vi "Interpret Driver Controls.vi"() -> ()   [LabVIEW 2018]
uses:
  Robot Global Data.vi
  SubSystems/Controllers/Driver Controller/Driver Controller Global.vi
  SubSystems/Drive Train/Drive Train Global.vi
  SubSystems/Lift/Lift Global.vi
  <vilib>/addons/control/pid/pid.llb/PID (DBL).vi
  SubSystems/Controllers/Manipulator Controlller/Manipulator Controller Global.vi
  SubSystems/HAB Climber/HAB Climber Global.vi
  SubSystems/Hatch Panel Intake/Hatch Panel Intake Global.vi
  SubSystems/Cargo Intake/Cargo Intake Global.vi
  <vilib>/addons/control/pid/NI_PID_pid.lvlib
panel:
  in  "Last Move Deadband":u32=500
  in  "Last Time Auto":u32=1171826
  in  "Camera Tracking":T1={"proportional gain (Kc)"=0.06, "integral time (Ti, min)"=0.0, "derivative time (Td, min)"=0.0}
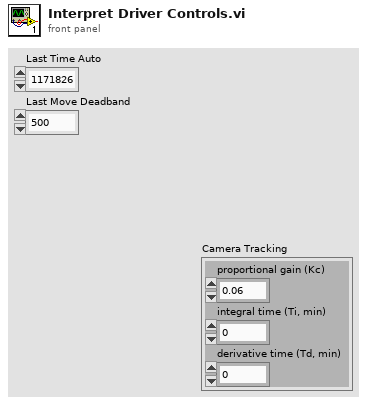
[diagram p1: front panel]
types:
  T1 = cluster{"proportional gain (Kc)":dbl, "integral time (Ti, min)":dbl, "derivative time (Td, min)":dbl}
  T2 = enum16{"Manual", "Hatch Panel Zone 1", "Hatch Panel Zone 2", "Hatch Panel Zone 3", "Cargo Zone 1", "Cargo Zone 2", "Cargo Zone 3", "Cargo Ship Zone"}
  T3 = cluster{"Rollover":dbl, "Yaw":dbl, "Cont Yaw":dbl}
  T4 = enum16{"Hatch Panel Zone 1", "Hatch Panel Zone 2", "Hatch Panel Zone 3", "Cargo Zone 1", "Cargo Zone 2", "Cargo Zone 3", "Cargo Ship Zone"}
  T5 = cluster{"offsetAngle H":dbl, "offsetAngle V":dbl, "area":dbl, "skew":dbl, "validTarget":dbl, "latency":dbl}
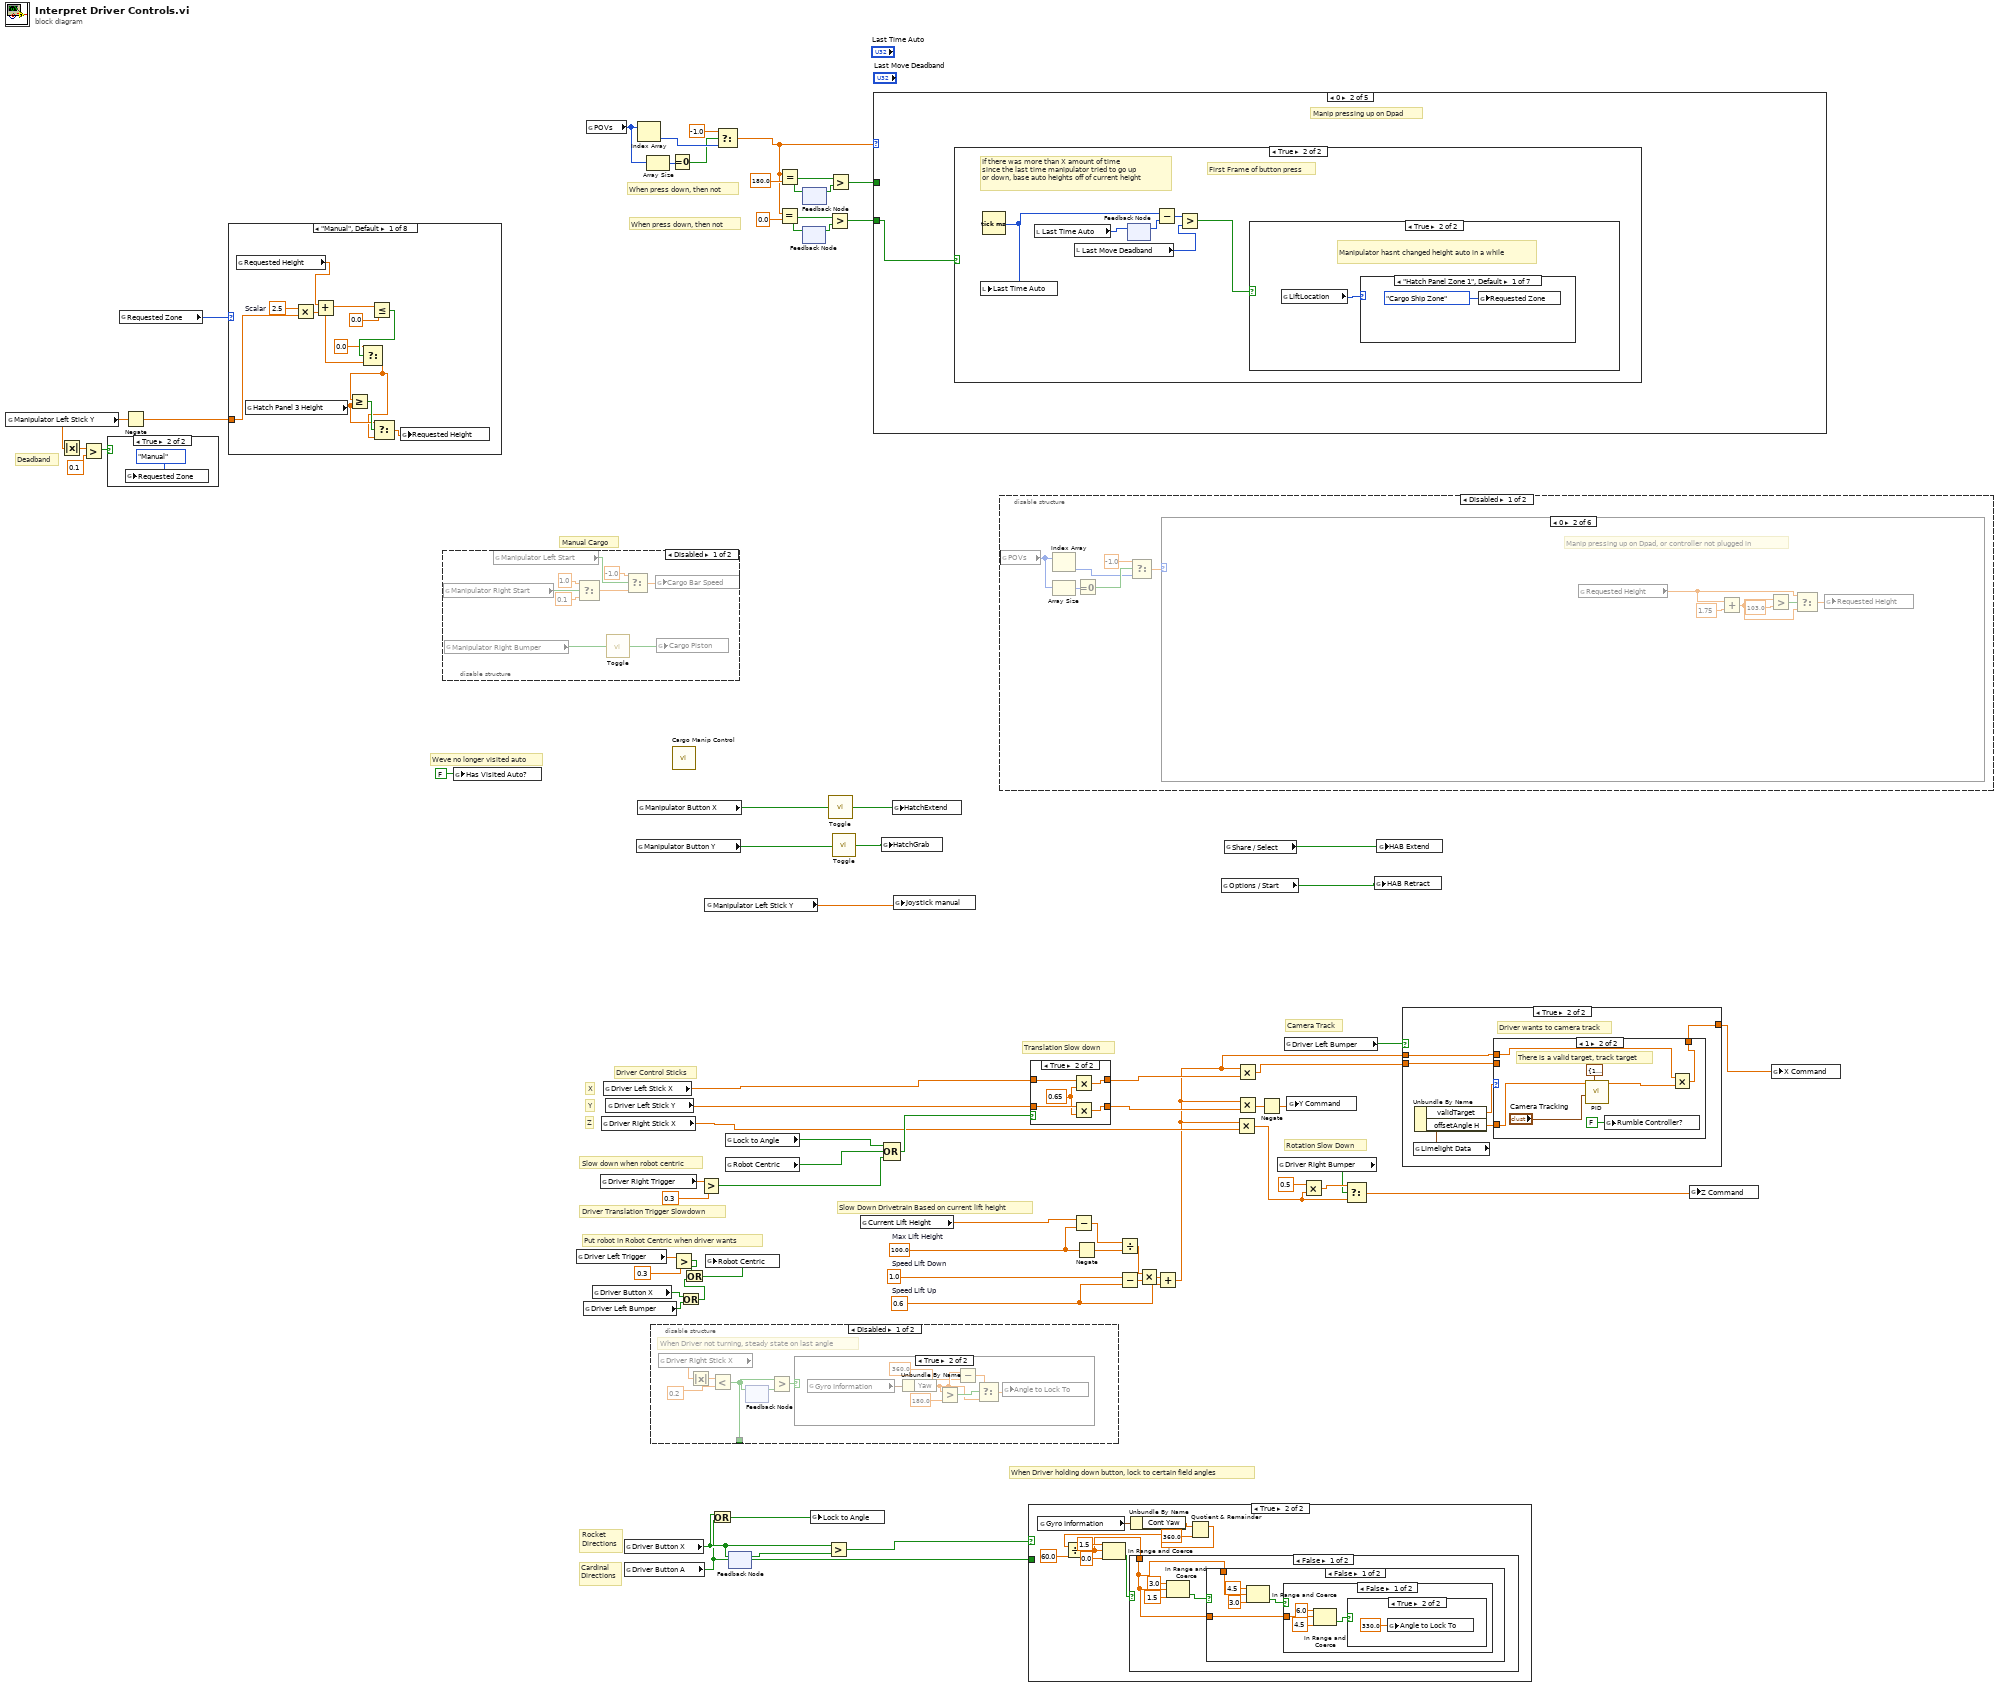
[diagram p0: block diagram]
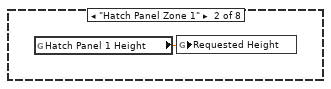
[diagram p3: hidden frame]
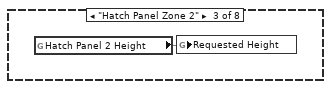
[diagram p4: hidden frame]
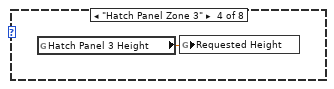
[diagram p5: hidden frame]
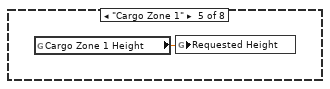
[diagram p6: hidden frame]
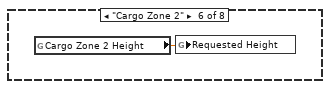
[diagram p7: hidden frame]
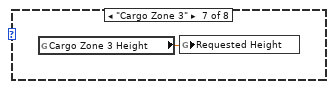
[diagram p8: hidden frame]
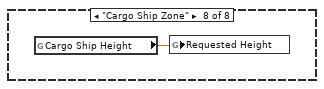
[diagram p9: hidden frame]
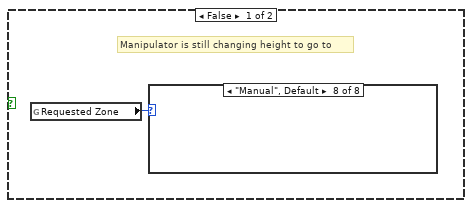
[diagram p12: hidden frame]
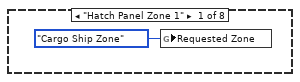
[diagram p13: hidden frame]
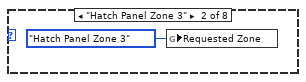
[diagram p14: hidden frame]
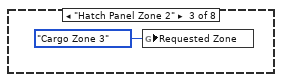
[diagram p15: hidden frame]
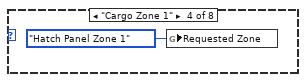
[diagram p16: hidden frame]
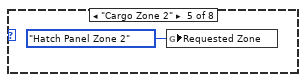
[diagram p17: hidden frame]
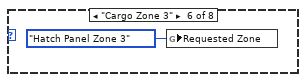
[diagram p18: hidden frame]
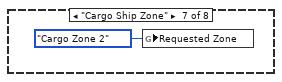
[diagram p19: hidden frame]
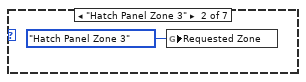
[diagram p20: hidden frame]
diagram:
  w51 = 0.6  # Speed Lift Up
  w55 = 1.0  # Speed Lift Down
  w49 = 100.0  # Max Lift Height
  # "When press down, then not"
  # "When press down, then not"
  # "Deadband"
  # "Manual Cargo"
  # "Weve no longer visited auto"
  # "Camera Track"
  # "Rotation Slow Down"
  # "Rocket\nDirections"
  # "Cardinal\nDirections"
  # "When Driver holding down button, lock to certain field angles"
  # "Slow Down Drivetrain Based on current lift height"
  # "Put robot in Robot Centric when driver wants"
  # "Slow down when robot centric"
  # "Driver Translation Trigger Slowdown"
  # "Translation Slow down"
  # "Z"
  # "Y"
  # "X"
  # "Driver Control Sticks"
  n1 = global read "Manipulator Controller Global.vi" "Manipulator Left Stick Y"() -> (w13:dbl)
  n2 = Absolute Value(x=w13) -> (abs(x)=w16:dbl)
  n3 = Greater?(x=w16, y=0.1) -> (0:w14:bool)
  n4 = case shown="True" w14 {
    frame False {
    }
    frame True {
      n5 = global write "Lift Global.vi" "Requested Zone"(T2."Manual" ("Requested Zone")) -> ()
    }
  }
  n6 = global read "Lift Global.vi" "Requested Zone"() -> (w17:T2)
  n7 = Negate(x=w13) -> (-x=w12:dbl)
  n8 = case shown="\"Manual\", Default" w17 {
    tunnel: w12 -> [w82 _ _ _ _ _ _ _]
    frame "Manual", Default {
      w81 = 2.5  # Scalar
      n9 = global read "Lift Global.vi" "Requested Height"() -> (w84:dbl)
      n10 = global read "Lift Global.vi" "Hatch Panel 3 Height"() -> (w75:dbl)
      n11 = Multiply(x=w81, y=w82) -> (x*y=w83:dbl)
      n12 = Add(x=w84, y=w83) -> (x+y=w77:dbl)
      n13 = Less Or Equal?(x=w77, y=0.0) -> (x <= y?=w79:bool)
      n14 = Select(t=0.0, s=w79, f=w77) -> (s? t:f=w74:dbl)
      n15 = Greater Or Equal?(x=w74, y=w75) -> (x >= y?=w76:bool)
      n16 = Select(t=w75, s=w76, f=w74) -> (s? t:f=w73:dbl)
      n17 = global write "Lift Global.vi" "Requested Height"(w73) -> ()
    }
    frame "Hatch Panel Zone 1" {
      n18 = global read "Lift Global.vi" "Hatch Panel 1 Height"() -> (w85:dbl)
      n19 = global write "Lift Global.vi" "Requested Height"(w85) -> ()
    }
    frame "Hatch Panel Zone 2" {
      n20 = global read "Lift Global.vi" "Hatch Panel 2 Height"() -> (w86:dbl)
      n21 = global write "Lift Global.vi" "Requested Height"(w86) -> ()
    }
    frame "Hatch Panel Zone 3" {
      n22 = global read "Lift Global.vi" "Hatch Panel 3 Height"() -> (w87:dbl)
      n23 = global write "Lift Global.vi" "Requested Height"(w87) -> ()
    }
    frame "Cargo Zone 1" {
      n24 = global read "Lift Global.vi" "Cargo Zone 1 Height"() -> (w88:dbl)
      n25 = global write "Lift Global.vi" "Requested Height"(w88) -> ()
    }
    frame "Cargo Zone 2" {
      n26 = global read "Lift Global.vi" "Cargo Zone 2 Height"() -> (w89:dbl)
      n27 = global write "Lift Global.vi" "Requested Height"(w89) -> ()
    }
    frame "Cargo Zone 3" {
      n28 = global read "Lift Global.vi" "Cargo Zone 3 Height"() -> (w90:dbl)
      n29 = global write "Lift Global.vi" "Requested Height"(w90) -> ()
    }
    frame "Cargo Ship Zone" {
      n30 = global read "Lift Global.vi" "Cargo Ship Height"() -> (w91:dbl)
      n31 = global write "Lift Global.vi" "Requested Height"(w91) -> ()
    }
  }
  n32 = disable-structure shown="Disabled" {
    frame Disabled {
      n33 = global read "Manipulator Controller Global.vi" "Manipulator Right Start"() -> (w97:bool)
      n34 = global read "Manipulator Controller Global.vi" "Manipulator Right Bumper"() -> (w100:bool)
      n35 = global read "Manipulator Controller Global.vi" "Manipulator Left Start"() -> (w96:bool)
      n36 = Select(t=1.0, s=w97, f=0.1) -> (s? t:f=w95:dbl)
      n37 = call "Toggle.vi"("Input"=w100) -> ("Output"=w99:bool)
      n38 = Select(t=-1.0, s=w96, f=w95) -> (s? t:f=w98:dbl)
      n39 = global write "Cargo Intake Global.vi" "Cargo Bar Speed"(w98) -> ()
      n40 = global write "Cargo Intake Global.vi" "Cargo Piston"(w99) -> ()
    }
    frame Enabled {
    }
  }
  n41 = global write "Robot Global Data.vi" "Has Visited Auto?"(FALSE ("Has Visited Auto?")) -> ()
  n42 = global read "Driver Controller Global.vi" "Driver Left Trigger"() -> (w68:dbl)
  n43 = global read "Driver Controller Global.vi" "Driver Left Bumper"() -> (w34:bool)
  n44 = global read "Manipulator Controller Global.vi" "POVs"() -> (w21:i16[])
  n45 = global read "Driver Controller Global.vi" "Driver Button X"() -> (w35:bool)
  n46 = global read "Driver Controller Global.vi" "Driver Right Trigger"() -> (w71:dbl)
  n47 = global read "Driver Controller Global.vi" "Driver Right Stick X"() -> (w22:dbl)
  n48 = global read "Driver Controller Global.vi" "Driver Left Stick X"() -> (w23:dbl)
  n49 = global read "Driver Controller Global.vi" "Driver Left Stick Y"() -> (w58:dbl)
  n50 = global read "Driver Controller Global.vi" "Driver Button X"() -> (w47:bool)
  n51 = global read "Driver Controller Global.vi" "Driver Button A"() -> (w45:bool)
  n52 = global read "Manipulator Controller Global.vi" "Manipulator Button Y"() -> (w33:bool)
  n53 = global read "Manipulator Controller Global.vi" "Manipulator Button X"() -> (w31:bool)
  n54 = Index Array(array=w21) -> (element=w18:i16)  [unwired: 1 in]
  n55 = Array Size(array=w21) -> (size(s)=w20:i32)
  n56 = disable-structure shown="Disabled" {
    disable-tunnel: [w101 _] -> _
    frame Disabled {
      # "When Driver not turning, steady state on last angle"
      n57 = global read "Driver Controller Global.vi" "Driver Right Stick X"() -> (w102:dbl)
      n58 = Absolute Value(x=w102) -> (abs(x)=w106:dbl)
      n59 = Less?(x=w106, y=0.2) -> (x < y?=w101:bool)
      n60 = feedback #1() -> (w104:bool)  [unwired: 1 in]
      n61 = feedback-in #1(w101) -> ()
      n62 = Greater?(x=w101, y=w104) -> (0:w103:bool)
      n63 = case shown="True" w103 {
        frame False {
        }
        frame True {
          n64 = global read "Drive Train Global.vi" "Gyro Information"() -> (w113:T3)
          n65 = Unbundle By Name(w113) -> ("Yaw"=w110:dbl)
          n66 = Greater?(x=w110, y=180.0) -> (0:w111:bool)
          n67 = Subtract(x=w110, y=360.0) -> (x-y=w108:dbl)
          n68 = Select(t=w108, s=w111, f=w110) -> (s? t:f=w107:dbl)
          n69 = global write "Drive Train Global.vi" "Angle to Lock To"(w107) -> ()
        }
      }
    }
    frame Enabled {
    }
  }
  n70 = Equal To 0?(x=w20) -> (x = 0?=w11:bool)
  n71 = call "Cargo Manip Control.vi"() -> ()  [unwired: 12 in]
  n72 = Greater?(x=w68, y=0.3) -> (0:w43:bool)
  n73 = Or(x=w35, y=w34) -> (x .or. y?=w36:bool)
  n74 = Or(x=w43, y=w36) -> (x .or. y?=w41:bool)
  n75 = Greater?(x=w71, y=0.3) -> (0:w63:bool)
  n76 = global read "Manipulator Controller Global.vi" "Manipulator Left Stick Y"() -> (w29:dbl)
  n77 = global write "Drive Train Global.vi" "Robot Centric"(w41) -> ()
  n78 = Or(x=w47, y=w45) -> (x .or. y?=w44:bool)
  n79 = Select(t=-1.0, s=w11, f=w18) -> (s? t:f=w3:dbl)
  n80 = global read "Drive Train Global.vi" "Lock to Angle"() -> (w42:bool)
  n81 = global read "Drive Train Global.vi" "Robot Centric"() -> (w62:bool)
  n82 = feedback #2() -> (w48:bool)  [unwired: 1 in]
  n83 = feedback-in #2(w47) -> ()
  n84 = Equal?(x=w3, y=0.0) -> (x = y?=w6:bool)
  n85 = Equal?(x=w3, y=180.0) -> (x = y?=w8:bool)
  n86 = feedback #3() -> (w5:bool)  [unwired: 1 in]
  n87 = feedback-in #3(w6) -> ()
  n88 = feedback-in #4(w8) -> ()
  n89 = feedback #4() -> (w9:bool)  [unwired: 1 in]
  n90 = global write "Drive Train Global.vi" "Lock to Angle"(w44) -> ()
  n91 = Greater?(x=w47, y=w48) -> (0:w46:bool)
  n92 = Greater?(x=w6, y=w5) -> (0:w2:bool)
  n93 = Greater?(x=w8, y=w9) -> (0:w7:bool)
  n94 = call "Toggle.vi"("Input"=w31) -> ("Output"=w32:bool)
  n95 = call "Toggle.vi"("Input"=w33) -> ("Output"=w30:bool)
  n96 = global read "Lift Global.vi" "Current Lift Height"() -> (w57:dbl)
  n97 = case shown="0" w3 {
    tunnel: w7 -> [_ _ w137 _ _]
    tunnel: w2 -> [_ w114 _ _ _]
    frame -1, Default {
      # "Nothing on the D-Pad is pressed!"
    }
    frame 0 {
      # "Manip pressing up on Dpad"
      n98 = case shown="True" w114 {
        frame False {
          # "Still pressing button, do nothing"
        }
        frame True {
          # "First Frame of button press"
          # "If there was more than X amount of time\nsince the last time manipulator tried to go up\nor down, base auto heights off of current height"
          n99 = Tick Count (ms)() -> (millisecond timer value=w117:u32)
          n100 = local write "Last Time Auto"(w117) -> ()
          n101 = local read "Last Time Auto"() -> (w116:u32)
          n102 = local read "Last Move Deadband"() -> (w118:u32)
          n103 = feedback #5() -> (w115:u32)  [unwired: 1 in]
          n104 = feedback-in #5(w116) -> ()
          n105 = Subtract(x=w117, y=w115) -> (x-y=w120:u32)
          n106 = Greater?(x=w120, y=w118) -> (0:w119:bool)
          n107 = case shown="True" w119 {
            frame False {
              # "Manipulator is still changing height to go to"
              n108 = global read "Lift Global.vi" "Requested Zone"() -> (w121:T2)
              n109 = case shown="\"Manual\", Default" w121 {
                frame "Hatch Panel Zone 1" {
                  n110 = global write "Lift Global.vi" "Requested Zone"(T2."Cargo Ship Zone" ("Requested Zone")) -> ()
                }
                frame "Hatch Panel Zone 3" {
                  n111 = global write "Lift Global.vi" "Requested Zone"(T2."Hatch Panel Zone 3" ("Requested Zone")) -> ()
                }
                frame "Hatch Panel Zone 2" {
                  n112 = global write "Lift Global.vi" "Requested Zone"(T2."Cargo Zone 3" ("Requested Zone")) -> ()
                }
                frame "Cargo Zone 1" {
                  n113 = global write "Lift Global.vi" "Requested Zone"(T2."Hatch Panel Zone 1" ("Requested Zone")) -> ()
                }
                frame "Cargo Zone 2" {
                  n114 = global write "Lift Global.vi" "Requested Zone"(T2."Hatch Panel Zone 2" ("Requested Zone")) -> ()
                }
                frame "Cargo Zone 3" {
                  n115 = global write "Lift Global.vi" "Requested Zone"(T2."Hatch Panel Zone 3" ("Requested Zone")) -> ()
                }
                frame "Cargo Ship Zone" {
                  n116 = global write "Lift Global.vi" "Requested Zone"(T2."Cargo Zone 2" ("Requested Zone")) -> ()
                }
                frame "Manual", Default {
                }
              }
            }
            frame True {
              # "Manipulator hasnt changed height auto in a while"
              n117 = global read "Lift Global.vi" "LiftLocation"() -> (w129:T4)
              n118 = case shown="\"Hatch Panel Zone 1\", Default" w129 {
                frame "Hatch Panel Zone 1", Default {
                  n119 = global write "Lift Global.vi" "Requested Zone"(T2."Cargo Ship Zone" ("Requested Zone")) -> ()
                }
                frame "Hatch Panel Zone 3" {
                  n120 = global write "Lift Global.vi" "Requested Zone"(T2."Hatch Panel Zone 3" ("Requested Zone")) -> ()
                }
                frame "Hatch Panel Zone 2" {
                  n121 = global write "Lift Global.vi" "Requested Zone"(T2."Cargo Zone 3" ("Requested Zone")) -> ()
                }
                frame "Cargo Zone 1" {
                  n122 = global write "Lift Global.vi" "Requested Zone"(T2."Hatch Panel Zone 1" ("Requested Zone")) -> ()
                }
                frame "Cargo Zone 2" {
                  n123 = global write "Lift Global.vi" "Requested Zone"(T2."Hatch Panel Zone 2" ("Requested Zone")) -> ()
                }
                frame "Cargo Zone 3" {
                  n124 = global write "Lift Global.vi" "Requested Zone"(T2."Hatch Panel Zone 3" ("Requested Zone")) -> ()
                }
                frame "Cargo Ship Zone" {
                  n125 = global write "Lift Global.vi" "Requested Zone"(T2."Cargo Zone 2" ("Requested Zone")) -> ()
                }
              }
            }
          }
        }
      }
    }
    frame 180 {
      # "Manip pressing down on Dpad"
      n126 = case shown="True" w137 {
        frame False {
          # "Still pressing button, do nothing"
        }
        frame True {
          # "First frame of button press"
          # "If there was more than X amount of time\nsince the last time manipulator tried to go up\nor down, base auto heights off of current height"
          n127 = Tick Count (ms)() -> (millisecond timer value=w142:u32)
          n128 = local write "Last Time Auto"(w142) -> ()
          n129 = local read "Last Time Auto"() -> (w139:u32)
          n130 = local read "Last Move Deadband"() -> (w141:u32)
          n131 = feedback #6() -> (w138:u32)  [unwired: 1 in]
          n132 = feedback-in #6(w139) -> ()
          n133 = Subtract(x=w142, y=w138) -> (x-y=w143:u32)
          n134 = Greater?(x=w143, y=w141) -> (0:w140:bool)
          n135 = case shown="False" w140 {
            frame False {
              # "Manipulator is still changing height to go to"
              n136 = global read "Lift Global.vi" "Requested Zone"() -> (w144:T2)
              n137 = case shown="\"Cargo Ship Zone\"" w144 {
                frame "Hatch Panel Zone 1" {
                  n138 = global write "Lift Global.vi" "Requested Zone"(T2."Cargo Zone 1" ("Requested Zone")) -> ()
                }
                frame "Hatch Panel Zone 3" {
                  n139 = global write "Lift Global.vi" "Requested Zone"(T2."Cargo Zone 3" ("Requested Zone")) -> ()
                }
                frame "Hatch Panel Zone 2" {
                  n140 = global write "Lift Global.vi" "Requested Zone"(T2."Cargo Zone 2" ("Requested Zone")) -> ()
                }
                frame "Cargo Zone 1" {
                  n141 = global write "Lift Global.vi" "Requested Zone"(T2."Cargo Zone 1" ("Requested Zone")) -> ()
                }
                frame "Cargo Zone 2" {
                  n142 = global write "Lift Global.vi" "Requested Zone"(T2."Cargo Ship Zone" ("Requested Zone")) -> ()
                }
                frame "Cargo Zone 3" {
                  n143 = global write "Lift Global.vi" "Requested Zone"(T2."Hatch Panel Zone 2" ("Requested Zone")) -> ()
                }
                frame "Cargo Ship Zone" {
                  n144 = global write "Lift Global.vi" "Requested Zone"(T2."Hatch Panel Zone 1" ("Requested Zone")) -> ()
                }
                frame "Manual", Default {
                }
              }
            }
            frame True {
              # "Manipulator hasnt changed height auto in a while"
              n145 = global read "Lift Global.vi" "LiftLocation"() -> (w152:T4)
              n146 = case shown="\"Hatch Panel Zone 1\", Default" w152 {
                frame "Hatch Panel Zone 1", Default {
                  n147 = global write "Lift Global.vi" "Requested Zone"(T2."Cargo Zone 1" ("Requested Zone")) -> ()
                }
                frame "Hatch Panel Zone 3" {
                  n148 = global write "Lift Global.vi" "Requested Zone"(T2."Cargo Zone 3" ("Requested Zone")) -> ()
                }
                frame "Hatch Panel Zone 2" {
                  n149 = global write "Lift Global.vi" "Requested Zone"(T2."Cargo Zone 2" ("Requested Zone")) -> ()
                }
                frame "Cargo Zone 1" {
                  n150 = global write "Lift Global.vi" "Requested Zone"(T2."Cargo Zone 1" ("Requested Zone")) -> ()
                }
                frame "Cargo Zone 2" {
                  n151 = global write "Lift Global.vi" "Requested Zone"(T2."Cargo Ship Zone" ("Requested Zone")) -> ()
                }
                frame "Cargo Zone 3" {
                  n152 = global write "Lift Global.vi" "Requested Zone"(T2."Hatch Panel Zone 2" ("Requested Zone")) -> ()
                }
                frame "Cargo Ship Zone" {
                  n153 = global write "Lift Global.vi" "Requested Zone"(T2."Hatch Panel Zone 1" ("Requested Zone")) -> ()
                }
              }
            }
          }
        }
      }
    }
    frame 90 {
      # "Go to Cargo in Cargo Ship Height"
      # "Right on D-Pad"
      n154 = global write "Lift Global.vi" "Requested Zone"(T2."Cargo Ship Zone" ("Requested Zone")) -> ()
    }
    frame 270 {
      # "Go to Hatch Level 1 Height"
      # "Left on D-Pad"
      n155 = global write "Lift Global.vi" "Requested Zone"(T2."Hatch Panel Zone 1" ("Requested Zone")) -> ()
    }
  }
  n156 = global write "Hatch Panel Intake Global.vi" "HatchGrab"(w30) -> ()
  n157 = Compound Arithmetic op=OR(w42, w62, w63) -> (w61:bool)
  n158 = global write "Hatch Panel Intake Global.vi" "HatchExtend"(w32) -> ()
  n159 = global write "Lift Global.vi" "Joystick manual"(w29) -> ()
  n160 = disable-structure shown="Disabled" {
    frame Disabled {
      n161 = global read "Manipulator Controller Global.vi" "POVs"() -> (w167:i16[])
      n162 = Index Array(array=w167) -> (element=w162:i16)  [unwired: 1 in]
      n163 = Array Size(array=w167) -> (size(s)=w166:i32)
      n164 = Equal To 0?(x=w166) -> (x = 0?=w164:bool)
      n165 = Select(t=-1.0, s=w164, f=w162) -> (s? t:f=w165:dbl)
      n166 = case shown="0" w165 {
        frame -1 {
          # "If the value changed (manip pressed button)\nchange set lift height to match"
          # "When button goes from\nnot pressed to pressed"
          n167 = global read "Manipulator Controller Global.vi" "Manipulator Square"() -> (w173:bool)
          n168 = feedback #7() -> (w174:bool)  [unwired: 1 in]
          n169 = feedback-in #7(w173) -> ()
          n170 = Greater?(x=w173, y=w174) -> (0:w170:bool)
          n171 = feedback #8() -> (w168:dbl)  [unwired: 1 in]
          n172 = feedback #9() -> (w172:dbl)  [unwired: 1 in]
          n173 = case shown="False" w170 {
            tunnel: [w184 w199] -> w169
            tunnel: w172 -> [w185 w198]
            frame False {
              # "When button goes from\nnot pressed to pressed"
              n174 = global read "Manipulator Controller Global.vi" "Manipulator Triangle"() -> (w187:bool)
              n175 = feedback #10() -> (w186:bool)  [unwired: 1 in]
              n176 = feedback-in #10(w187) -> ()
              n177 = Greater?(x=w187, y=w186) -> (0:w183:bool)
              n178 = case shown="True" w183 {
                tunnel: w185 -> [w188 w190]
                tunnel: [w188 w192] -> w184
                frame False {
                }
                frame True {
                  # "If counter smaller than 5\nadd 1"
                  n179 = Less?(x=w190, y=5.0) -> (x < y?=w189:bool)
                  n180 = case shown="True" w189 {
                    tunnel: [w193 w195] -> w192
                    tunnel: w190 -> [w193 w194]
                    frame False {
                    }
                    frame True {
                      n181 = Increment(x=w194) -> (x+1=w195:dbl)
                    }
                  }
                }
              }
            }
            frame True {
              # "If counter bigger than 0\nsubtract 1"
              n182 = Greater?(x=w198, y=0.0) -> (0:w197:bool)
              n183 = case shown="False" w197 {
                tunnel: [0.0 ("y") w202] -> w199
                tunnel: w198 -> [_ w201]
                frame False {
                }
                frame True {
                  n184 = Decrement(x=w201) -> (x-1=w202:dbl)
                }
              }
            }
          }
          n185 = feedback-in #8(w169) -> ()
          n186 = Not Equal?(x=w169, y=w168) -> (x != y?=w171:bool)
          n187 = case shown="True" w171 {
            tunnel: w169 -> [_ w175]
            frame False {
              # "Manipulator didnt request change"
            }
            frame True {
              # "Set height request to new value"
              n188 = case shown="0, Default" w175 {
                tunnel: [w177 w178 w179 w180 w181 w182] -> w176
                frame 0, Default {
                  n189 = global read "Lift Global.vi" "Cargo Zone 1 Height"() -> (w177:dbl)
                }
                frame 1 {
                  n190 = global read "Lift Global.vi" "Hatch Panel 1 Height"() -> (w178:dbl)
                }
                frame 2 {
                  n191 = global read "Lift Global.vi" "Cargo Zone 2 Height"() -> (w179:dbl)
                }
                frame 3 {
                  n192 = global read "Lift Global.vi" "Hatch Panel 2 Height"() -> (w180:dbl)
                }
                frame 4 {
                  n193 = global read "Lift Global.vi" "Cargo Zone 3 Height"() -> (w181:dbl)
                }
                frame 5 {
                  n194 = global read "Lift Global.vi" "Hatch Panel 3 Height"() -> (w182:dbl)
                }
              }
              n195 = global write "Lift Global.vi" "Requested Height"(w176) -> ()
            }
          }
          n196 = global write "Lift Global.vi" "Lift Auto Position"(w169) -> ()
          n197 = feedback-in #9(w169) -> ()
        }
        frame 0 {
          # "Manip pressing up on Dpad, or controller not plugged in"
          n198 = global read "Lift Global.vi" "Requested Height"() -> (w204:dbl)
          n199 = Add(x=w204, y=1.75) -> (x+y=w203:dbl)
          n200 = Greater?(x=w203, y=103.0) -> (0:w205:bool)
          n201 = Select(t=w204, s=w205, f=w203) -> (s? t:f=w206:dbl)
          n202 = global write "Lift Global.vi" "Requested Height"(w206) -> ()
        }
        frame 180 {
          # "Manip pressing down on Dpad"
          n203 = global read "Lift Global.vi" "Requested Height"() -> (w209:dbl)
          n204 = Add(x=w209, y=-1.0) -> (x+y=w211:dbl)
          n205 = Less?(x=w211, y=0.0) -> (x < y?=w212:bool)
          n206 = Select(t=w209, s=w212, f=w211) -> (s? t:f=w210:dbl)
          n207 = global write "Lift Global.vi" "Requested Height"(w210) -> ()
        }
        frame 90 {
          # "Go to Cargo in Cargo Ship Height"
          # "Right on D-Pad"
          n208 = global read "Lift Global.vi" "Cargo Ship Height"() -> (w215:dbl)
          n209 = global write "Lift Global.vi" "Requested Height"(w215) -> ()
        }
        frame 270 {
          # "Go to Hatch Level 1 Height"
          # "Left on D-Pad"
          n210 = global read "Lift Global.vi" "Hatch Panel 1 Height"() -> (w216:dbl)
          n211 = global write "Lift Global.vi" "Requested Height"(w216) -> ()
        }
        frame -100, Default {
        }
      }
    }
    frame Enabled {
    }
  }
  n212 = case shown="True" w46 {
    tunnel: w45 -> [w218 _]
    frame False {
      n213 = feedback #11() -> (w219:bool)  [unwired: 1 in]
      n214 = feedback-in #11(w218) -> ()
      n215 = Greater?(x=w218, y=w219) -> (0:w217:bool)
      n216 = case shown="True" w217 {
        frame False {
        }
        frame True {
          n217 = global read "Drive Train Global.vi" "Gyro Information"() -> (w226:T3)
          n218 = Unbundle By Name(w226) -> ("Yaw"=w223:dbl)
          n219 = Add(x=w223, y=180.0) -> (x+y=w222:dbl)
          n220 = Divide(x=w222, y=90.0) -> (x/y=w224:dbl)
          n221 = Round To Nearest(number=w224) -> (nearest integer value=w220:dbl)
          n222 = case shown="1" w220 {
            frame 0, Default {
              n223 = global write "Drive Train Global.vi" "Angle to Lock To"(180.0 ("Angle to Lock To")) -> ()
            }
            frame 1 {
              n224 = global write "Drive Train Global.vi" "Angle to Lock To"(270.0 ("Angle to Lock To")) -> ()
            }
            frame 2 {
              n225 = global write "Drive Train Global.vi" "Angle to Lock To"(0.0 ("Angle to Lock To")) -> ()
            }
            frame 3 {
              n226 = global write "Drive Train Global.vi" "Angle to Lock To"(90.0 ("Angle to Lock To")) -> ()
            }
            frame 4 {
              n227 = global write "Drive Train Global.vi" "Angle to Lock To"(180.0 ("Angle to Lock To")) -> ()
            }
          }
        }
      }
    }
    frame True {
      n228 = global read "Drive Train Global.vi" "Gyro Information"() -> (w240:T3)
      n229 = Unbundle By Name(w240) -> ("Cont Yaw"=w238:dbl)
      n230 = Quotient & Remainder(x=w238, y=360.0) -> (x-y*floor(x/y)=w236:dbl)  [unwired: 1 out]
      n231 = Divide(x=w236, y=60.0) -> (x/y=w232:dbl)
      n232 = In Range and Coerce(upper limit=1.5, x=w232, lower limit=0.0) -> (In Range?=w233:bool)  [unwired: 1 out]
      n233 = case shown="False" w233 {
        tunnel: w232 -> [w241 _]
        frame False {
          n234 = In Range and Coerce(upper limit=3.0, x=w241, lower limit=1.5) -> (In Range?=w242:bool)  [unwired: 1 out]
          n235 = case shown="False" w242 {
            tunnel: w241 -> [w247 _]
            tunnel: w241 -> [w245 _]
            frame False {
              n236 = In Range and Coerce(upper limit=4.5, x=w247, lower limit=3.0) -> (In Range?=w246:bool)  [unwired: 1 out]
              n237 = case shown="False" w246 {
                tunnel: w245 -> [w251 _]
                frame False {
                  n238 = In Range and Coerce(upper limit=6.0, x=w251, lower limit=4.5) -> (In Range?=w250:bool)  [unwired: 1 out]
                  n239 = case shown="True" w250 {
                    frame False {
                    }
                    frame True {
                      n240 = global write "Drive Train Global.vi" "Angle to Lock To"(330.0 ("Angle to Lock To")) -> ()
                    }
                  }
                }
                frame True {
                  n241 = global write "Drive Train Global.vi" "Angle to Lock To"(210.0 ("Angle to Lock To")) -> ()
                }
              }
            }
            frame True {
              n242 = global write "Drive Train Global.vi" "Angle to Lock To"(150.0 ("Angle to Lock To")) -> ()
            }
          }
        }
        frame True {
          n243 = global write "Drive Train Global.vi" "Angle to Lock To"(30.0 ("Angle to Lock To")) -> ()
        }
      }
    }
  }
  n244 = case shown="True" w61 {
    tunnel: w58 -> [w259 w264]
    tunnel: [w259 w263] -> w60
    tunnel: [w258 w262] -> w59
    tunnel: w23 -> [w258 w261]
    frame False {
    }
    frame True {
      w260 = 0.65 ("Y Slower")
      n245 = Multiply(x=w261, y=w260) -> (x*y=w262:dbl)
      n246 = Multiply(x=w264, y=w260) -> (x*y=w263:dbl)
    }
  }
  n247 = Subtract(x=w57, y=w49) -> (x-y=w56:dbl)
  n248 = Negate(x=w49) -> (-x=w50:dbl)
  n249 = Divide(x=w56, y=w50) -> (x/y=w54:dbl)
  n250 = Subtract(x=w55, y=w51) -> (x-y=w53:dbl)
  n251 = Multiply(x=w54, y=w53) -> (x*y=w52:dbl)
  n252 = Add(x=w52, y=w51) -> (x+y=w1:dbl)
  n253 = global read "Manipulator Controller Global.vi" "Options / Start"() -> (w27:bool)
  n254 = global read "Manipulator Controller Global.vi" "Share / Select"() -> (w28:bool)
  n255 = Multiply(x=w1, y=w22) -> (x*y=w67:dbl)
  n256 = Multiply(x=w1, y=w59) -> (x*y=w38:dbl)
  n257 = Multiply(x=w1, y=w60) -> (x*y=w26:dbl)
  n258 = Negate(x=w26) -> (-x=w25:dbl)
  n259 = global read "Driver Controller Global.vi" "Driver Right Bumper"() -> (w64:bool)
  n260 = global read "Driver Controller Global.vi" "Driver Left Bumper"() -> (w40:bool)
  n261 = global write "Drive Train Global.vi" "Y Command"(w25) -> ()
  n262 = Multiply(x=0.5, y=w67) -> (x*y=w66:dbl)
  n263 = Select(t=w66, s=w64, f=w67) -> (s? t:f=w39:dbl)
  n264 = global write "HAB Climber Global.vi" "HAB Retract"(w27) -> ()
  n265 = global write "HAB Climber Global.vi" "HAB Extend"(w28) -> ()
  n266 = case shown="True" w40 {
    tunnel: w38 -> [w266 w270]
    tunnel: [w266 w268] -> w37
    tunnel: w1 -> [_ w267]
    frame False {
      # "Driver not attepting to camera track, be normal"
      n267 = global write "Driver Controller Global.vi" "Rumble Controller?"(FALSE ("Rumble Controller?")) -> ()
    }
    frame True {
      # "Driver wants to camera track"
      n268 = global read "Robot Global Data.vi" "Limelight Data"() -> (w272:T5)
      n269 = Unbundle By Name(w272) -> ("validTarget"=w271:dbl, "offsetAngle H"=w269:dbl)
      n270 = case shown="1" w271 {
        tunnel: w270 -> [w273 _]
        tunnel: w269 -> [_ w278]
        tunnel: [w273 w277] -> w268
        tunnel: w267 -> [_ w275]
        frame 0, Default {
          # "No Valid Target, keep using driver controls\nand rumble controller so knows not tracking"
          n271 = global write "Driver Controller Global.vi" "Rumble Controller?"(TRUE ("Rumble Controller?")) -> ()
        }
        frame 1 {
          # "There is a valid target, track target"
          n272 = call-poly <vilib>:"PID.vi"("output range"=cluster{"output high":dbl, "output low":dbl} {"output high"=1.0, "output low"=-1.0}, "PID gains"="Camera Tracking", "setpoint"=w278) -> ("output"=w276:dbl)  [unwired: 7 in, 1 out]
          n273 = global write "Driver Controller Global.vi" "Rumble Controller?"(FALSE ("Rumble Controller?")) -> ()
          n274 = Multiply(x=w275, y=w276) -> (x*y=w277:dbl)
        }
      }
    }
  }
  n275 = global write "Drive Train Global.vi" "Z Command"(w39) -> ()
  n276 = global write "Drive Train Global.vi" "X Command"(w37) -> ()
